vi "Config Horiz.vi"(6 "Record Sample Length":i32(ring)=2 items=["500 points", "1000 points", "2500 points", "5000 points", "15000 points", "50000 points", "75000 points", "100000 points", "130000 points", "250000 points", "500000 points"], 7 "error in (no error)":errorcluster, 8 "Horizontle Trace Display":i32(ring)=1 items=["Main Only", "Intensified", "Delayed Only"], 9 "Horizontle Scale":i32(ring)=19 items=["100ps/div", "200ps/div", "500ps/div", "1ns/div", "2ns/div", "5ns/div", "10ns/div", "20ns/div", "50ns/div", "100ns/div", "200ns/div", "500ns/div", "1µs/div", "2µs/div", "5µs/div", "10µs/div", "20µs/div", "50µs/div", "100µs/div", "200µs/div", "500µs/div", "1ms/div", "2ms/div", "5ms/div", "10ms/div", "20ms/div", "50ms/div", "100ms/div", "200ms/div", "500ms/div", "1s/div", "2s/div", "5s/div", "10s/div"], 10 "Scope Address":refnum<visa-resource-name>) -> (0 "error out":errorcluster, 3 "reference out":refnum<visa-resource-name>)   [LabVIEW 2020]
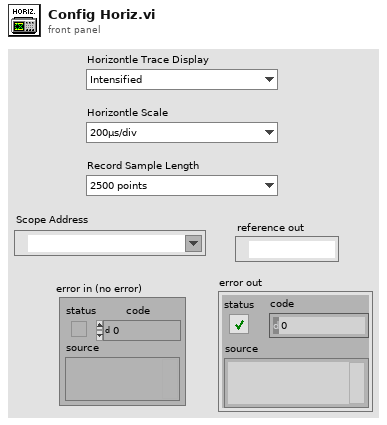
[diagram p1: front panel]
types:
  T1 = cluster{"delay mode (runs after:0)":i32, "delay scaling (50micros/div:16)":i32, "delay events (2)":ext, "delay by (time:0)":i32, "delay time (16.0E-9)":ext}
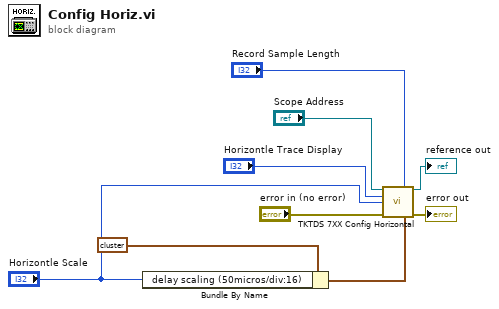
[diagram p0: block diagram]
diagram:
  n1 = Bundle By Name(cluster=T1 {"delay mode (runs after:0)"=0, "delay scaling (50micros/div:16)"=18, "delay events (2)"=2.0, "delay by (time:0)"=0, "delay time (16.0E-9)"=1.6e-08}, "delay scaling (50micros/div:16)"="Horizontle Scale") -> (w5:T1)
  n2 = call <instrlib>:"TKTDS 7XX Config Horizontal.vi"("VISA session"="Scope Address", "record length (500:0)"="Record Sample Length", "horizontal mode\n(main only:0)"="Horizontle Trace Display", "main scaling\n(500ps:1)"="Horizontle Scale", "error in (no error)"="error in (no error)", 14:w5) -> ("dup VISA session"=→"reference out":refnum<visa-resource-name>, "error out"=→"error out":errorcluster)  [unwired: 8 in]
